vi "Calculate CPR.vi"(5 "steps":i32, 7 "phase range":i32, 8 "error in (no error)":errorcluster, 11 "path in":path) -> (0 "error out":errorcluster, 3 "output Plot":T1)   [LabVIEW 2023]
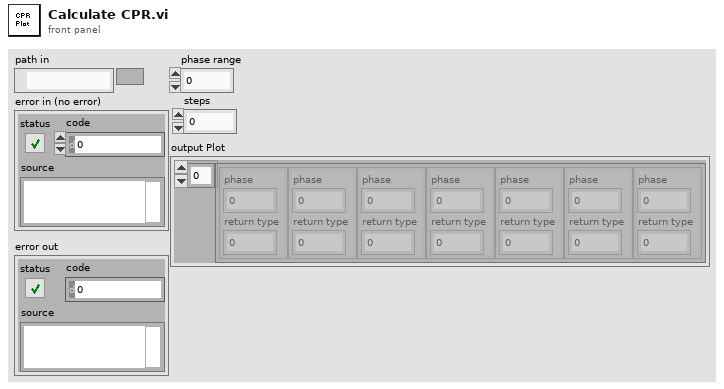
[diagram p1: front panel]
types:
  T1 = cluster{cluster{"phase":dbl, "return type":dbl}[]}
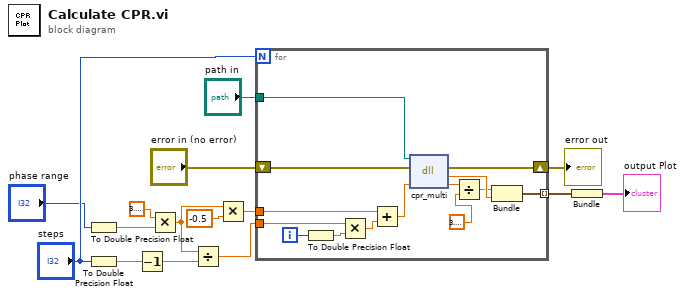
[diagram p0: block diagram]
diagram:
  n1 = To Double Precision Float(number="phase range") -> (double precision float=w6:dbl)
  n2 = To Double Precision Float(number="steps") -> (double precision float=w12:dbl)
  n3 = Decrement(x=w12) -> (x-1=w11:dbl)
  n4 = Multiply(x=3.141592653589793, y=w6) -> (x*y=w1:dbl)
  n5 = Divide(x=w1, y=w11) -> (x/y=w9:dbl)
  n6 = Multiply(x=w1, y=-0.5) -> (x*y=w4:dbl)
  n7 = for {
    N: "steps" -> [_]
    tunnel: "path in" -> [w29]
    shift-right: [w27] -> w13
    shift-left: "error in (no error)" -> [w28]
    tunnel: w9 -> [w25]
    tunnel: w4 -> [w22]
    tunnel: [w18] -> w3 mode=indexing
    i -> [w26]
    n8 = To Double Precision Float(number=w26) -> (double precision float=w24:dbl)
    n9 = Multiply(x=w25, y=w24) -> (x*y=w23:dbl)
    n10 = Add(x=w22, y=w23) -> (x+y=w21:dbl)
    n11 = dll-call lib="C:/Users/yg/Box/Guang Yue uiuc research box folder/computation/S-TI-S jj simulation c/Release/ygDLL.dll" fn="cpr_multi"(path in=w29, error in=w28, "phase"=w21) -> (error out=w27:errorcluster, "return type"=w19:dbl, "phase"=w20:dbl)  [unwired: 1 in, 1 out]
    n12 = Divide(x=w20, y=3.141592653589793) -> (x/y=w17:dbl)
    n13 = Bundle(w17, "return type"=w19) -> (w18:cluster{dbl, "return type":dbl})  [unwired: 1 in]
  }
  "error out" <- w13
  n14 = Bundle(w3) -> (→"output Plot":cluster{cluster{dbl, "return type":dbl}[]})  [unwired: 1 in]
